vi "Read write operation timeout.vi"(8 "error in (no error)":errorcluster, 11 "SMSD ADU in":refnum<class "SMSD ADU.lvclass">) -> (0 "error out":errorcluster, 2 "write operation timeout":u32=100, 3 "SMSD ADU out":refnum<class "SMSD ADU.lvclass">)   [LabVIEW 2021, in "SMSD ADU.lvclass"]
uses:
  SMSD ADU.lvclass
  SMSD ADU.lvclass/SMSD ADU.ctl
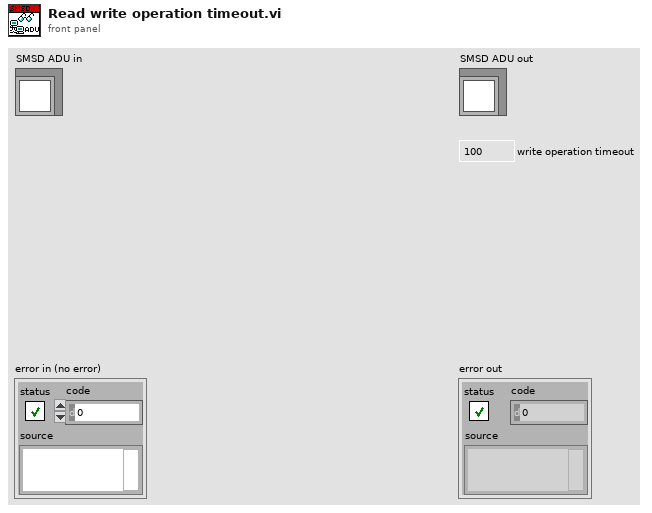
[diagram p1: front panel]
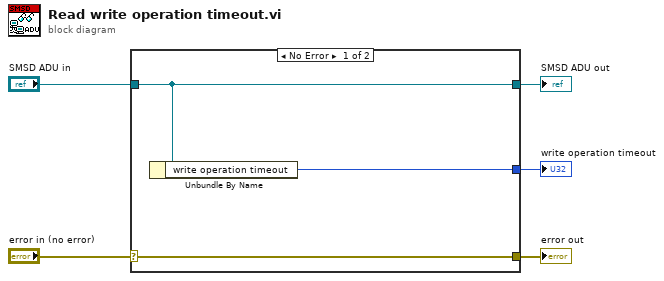
[diagram p0: block diagram]
diagram:
  n1 = case shown="No Error" "error in (no error)" {
    selector: "error in (no error)" -> [w8 w9]
    tunnel: [w8 w9] -> w4
    tunnel: [w7 w10] -> w2
    tunnel: "SMSD ADU in" -> [w7 w10]
    tunnel: [w6 _] -> w1
    frame No Error {
      n2 = Unbundle By Name(w7) -> ("write operation timeout"=w6:u32)
    }
    frame Error {
    }
  }
  "error out" <- w4
  "SMSD ADU out" <- w2
  "write operation timeout" <- w1
